vi "Create.vi"(8 "error in (no error)":errorcluster, 10 "Variable Interlocks":string[](array[string]), 11 "Variable Names":string[](array[string])) -> (0 "error out":errorcluster, 3 "Interlocks":T1[](array[typedef]))   [LabVIEW 2022 SP3, in "Interlocks.lvlib"]
uses:
  Interlocks.lvlib
  Controls/Interlock.ctl
  Controls/Token Type.ctl
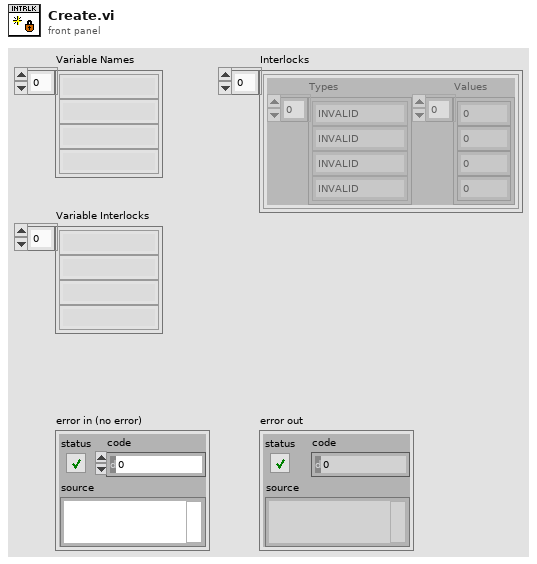
[diagram p1: front panel]
types:
  T1 = typedef "Interlocks.lvlib/Interlock.ctl" = cluster{"Types":T2[], "Values":dbl[]}
  T2 = typedef "Interlocks.lvlib/Token Type.ctl" = enum8{"INVALID", "NOT", "AND", "OR", "EE", "NE", "LT", "GT", "LTE", "GTE", "PLUS", "MINUS", "MULTIPLY", "DIVIDE", "MODULUS", "LPAREN", "RPAREN", "LITERAL", "IDENTIFIER", "DEFINITION"}
  T3 = typedef "Interlocks.lvlib/Token.ctl" = cluster{"Offset":i32, "Type":T2, "Value":string}
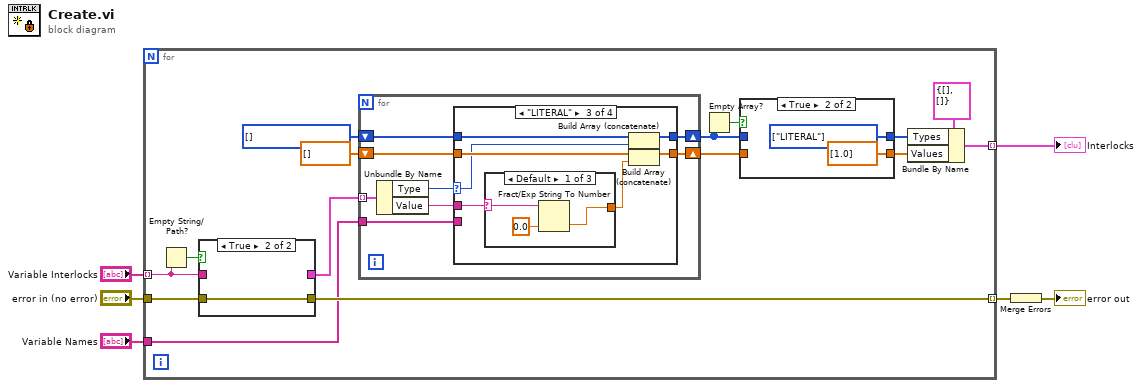
[diagram p0: block diagram]
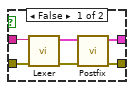
[diagram p3: hidden frame]
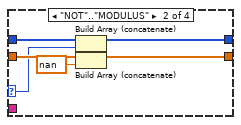
[diagram p5: hidden frame]
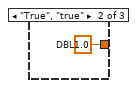
[diagram p6: hidden frame]
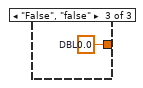
[diagram p7: hidden frame]
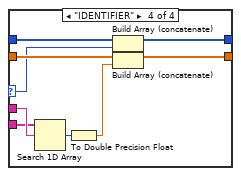
[diagram p8: hidden frame]
diagram:
  n1 = for {
    tunnel: "Variable Names" -> [w18]
    tunnel: [w19] -> w2 mode=indexing
    tunnel: "error in (no error)" -> [w17]
    tunnel: [w21] -> w5 mode=indexing
    tunnel: "Variable Interlocks" -> [w16] mode=indexing
    w14 = T2[] [] items=["INVALID", "NOT", "AND", "OR", "EE", "NE", "LT", "GT", "LTE", "GTE", "PLUS", "MINUS", "MULTIPLY", "DIVIDE", "MODULUS", "LPAREN", "RPAREN", "LITERAL", "IDENTIFIER", "DEFINITION"]
    n2 = Empty String/Path?(string/path=w16) -> (empty?=w12:bool)
    n3 = case shown="True" w12 {
      tunnel: [w31 w32] -> w21
      tunnel: w17 -> [w30 w32]
      tunnel: w16 -> [w29 _]
      tunnel: [w26 _] -> w15
      frame False {
        n4 = call "Lexer.vi"("error in (no error)"=w30, "Input"=w29) -> ("error out"=w28:errorcluster, "Tokens"=w27:T3[])  [unwired: 8 in]
        n5 = call "Postfix.vi"("error in (no error)"=w28, "Infix"=w27) -> ("error out"=w31:errorcluster, "Postfix"=w26:T3[])  [unwired: 8 in]
      }
      frame True {
      }
    }
    n6 = for {
      tunnel: w15 -> [w40] mode=indexing
      shift-right: [w38] -> w10
      shift-left: w14 -> [w37]
      shift-right: [w35] -> w7
      shift-left: dbl[] [] ("Values") -> [w36]
      tunnel: w18 -> [w33]
      n7 = Unbundle By Name(w40) -> ("Type"=w39:T2, "Value"=w34:string)
      n8 = case shown="\"LITERAL\"" w39 {
        selector: w39 -> [_ w44 w51 w65]
        tunnel: [w42 w46 w53 w67] -> w38
        tunnel: w37 -> [w42 w48 w55 w69]
        tunnel: w36 -> [w41 w47 w54 w68]
        tunnel: [w41 w45 w52 w66] -> w35
        tunnel: w34 -> [_ _ w50 w64]
        tunnel: w33 -> [_ _ _ w63]
        frame "INVALID", "LPAREN", "RPAREN", "DEFINITION" {
        }
        frame "NOT".."MODULUS" {
          n9 = Build Array (concatenate)(w48, w44) -> (w46:T2[])
          n10 = Build Array (concatenate)(w47, nan) -> (w45:dbl[])
        }
        frame "LITERAL" {
          n11 = case shown="Default" w50 {
            selector: w50 -> [w58 _ _]
            tunnel: [w56 w59 w60] -> w49
            frame Default {
              n12 = Fract/Exp String To Number(string=w58, default (0 dbl)=0.0 ("DBL")) -> (number=w56:dbl)  [unwired: 2 in, 1 out]
            }
            frame "True", "true" {
              w59 = 1.0  # DBL
            }
            frame "False", "false" {
              w60 = 0.0  # DBL
            }
          }
          n13 = Build Array (concatenate)(w55, w51) -> (w53:T2[])
          n14 = Build Array (concatenate)(w54, w49) -> (w52:dbl[])
        }
        frame "IDENTIFIER" {
          n15 = Search 1D Array(1D array=w63, element=w64) -> (index of element=w62:i32)  [unwired: 1 in]
          n16 = To Double Precision Float(number=w62) -> (double precision float=w61:dbl)
          n17 = Build Array (concatenate)(w69, w65) -> (w67:T2[])
          n18 = Build Array (concatenate)(w68, w61) -> (w66:dbl[])
        }
      }
    }
    n19 = Empty Array?(array=w10) -> (empty?=w9:bool)
    n20 = case shown="True" w9 {
      tunnel: [w23 w25] -> w11
      tunnel: w10 -> [w23 _]
      tunnel: [w22 dbl[] [1.0] ("Values")] -> w8
      tunnel: w7 -> [w22 _]
      frame False {
      }
      frame True {
        w25 = T2[] [enum."LITERAL"] items=["INVALID", "NOT", "AND", "OR", "EE", "NE", "LT", "GT", "LTE", "GTE", "PLUS", "MINUS", "MULTIPLY", "DIVIDE", "MODULUS", "LPAREN", "RPAREN", "LITERAL", "IDENTIFIER", "DEFINITION"]
      }
    }
    n21 = Bundle By Name(cluster=T1 {"Types"=[], "Values"=[]} ("Definition"), "Types"=w11, "Values"=w8) -> (w19:T1)
  }
  "Interlocks" <- w2
  n22 = Merge Errors(w5) -> (→"error out":errorcluster)
